vi "Initialize.vi"(8 "error in (no error)":errorcluster, 11 "VISA in":refnum<class "VISA.lvclass">) -> (0 "error out":errorcluster, 3 "VISA out":refnum<class "VISA.lvclass">)   [LabVIEW 2013, in "Protocol Classes.lvlib" / "VISA.lvclass"]
uses:
  VISA.lvclass
  VISA.lvclass/VISA.ctl
  Read VISA Resource.vi
  Read Enable Termination Character.vi
  Read Termination Character.vi
  Read Timeout.vi
  Write Ref.vi
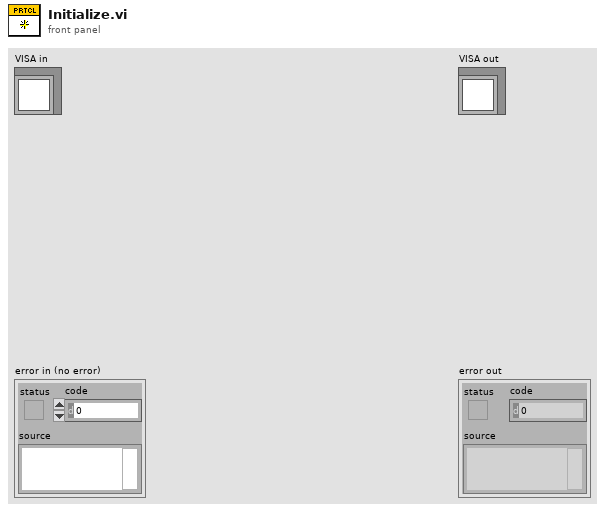
[diagram p1: front panel]
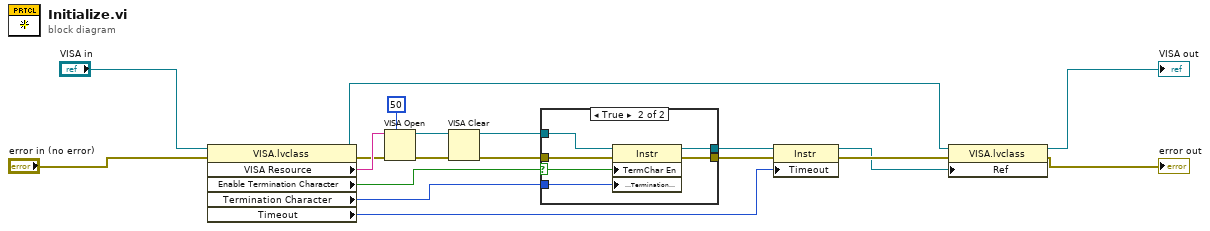
[diagram p0: block diagram]
diagram:
  n1 = property class="VISA.lvclass"(reference="VISA in", error in="error in (no error)") -> (reference out=w16:refnum<class "VISA.lvclass">, error out=w17:errorcluster, "VISA Resource"=w19:string, "Enable Termination Character"=w9:bool, "Termination Character"=w8:u8, "Timeout"=w1:u32)
  n2 = VISA Open(timeout (0)=u32 50 ("VISA Open timeout (0)"), error in (no error)=w17, VISA resource name=w19) -> (VISA resource name=w15:refnum<visa-resource-name>, error out=w14:errorcluster)  [unwired: 2 in]
  n3 = VISA Clear(VISA resource name=w15, error in (no error)=w14) -> (VISA resource name out=w10:refnum<visa-resource-name>, error out=w11:errorcluster)
  n4 = case shown="True" w9 {
    selector: w9 -> [_ w22]
    tunnel: w10 -> [w20 w27]
    tunnel: w11 -> [w21 w26]
    tunnel: [w20 w25] -> w2
    tunnel: [w21 w24] -> w5
    tunnel: w8 -> [_ w23]
    frame False {
    }
    frame True {
      n5 = property class="Instr"(reference=w27, error in=w26, "TermChar En"=w22, "Message Based Settings:Termination Character"=w23) -> (reference out=w25:refnum<visa-resource-name>, error out=w24:errorcluster)
    }
  }
  n6 = property class="Instr"(reference=w2, error in=w5, "Timeout"=w1) -> (reference out=w3:refnum<visa-resource-name>, error out=w4:errorcluster)
  n7 = property class="VISA.lvclass"(reference=w16, error in=w4, "Ref"=w3) -> (reference out=→"VISA out":refnum<class "VISA.lvclass">, error out=→"error out":errorcluster)
